vi "ViewAnalysisResults.vi"(7 "LabVIEW Web Service Request":refnum<class "Web Request.lvclass">) -> (3 "Data":T1[](array[typedef]))   [LabVIEW 2019]
uses:
  <vilib>/wsapi/Web Request.lvclass
  ParameterData.ctl
panel:
  # "Use the Web Service Request input terminal to call the VIs on the Web Services palette. Do not remove it from the connector pane unless you don't need access to the palette."
  # "Each additional control wired to the connector pane will be available as an input in the URL. To include an indicator in terminal-mode output (the default setting), it must also be wired to the connector pane."
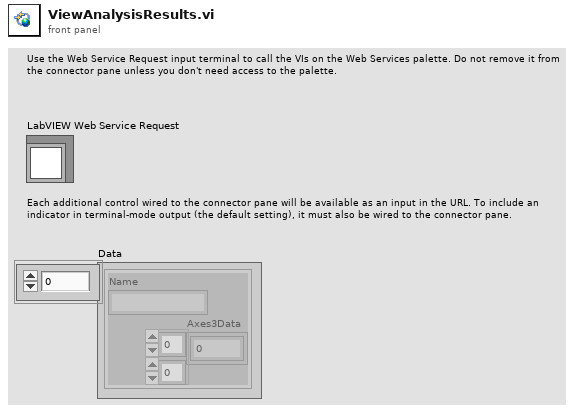
[diagram p1: front panel]
types:
  T1 = typedef "ParameterData.ctl" = cluster{"Name":string, "Axes3Data":dbl[][]}
  T2 = enum16{"open", "open or create", "create or replace", "create", "open (read-only)"}
  T3 = enum16{"open", "replace", "create", "open or create", "replace or create", "replace or create with confirmation"}
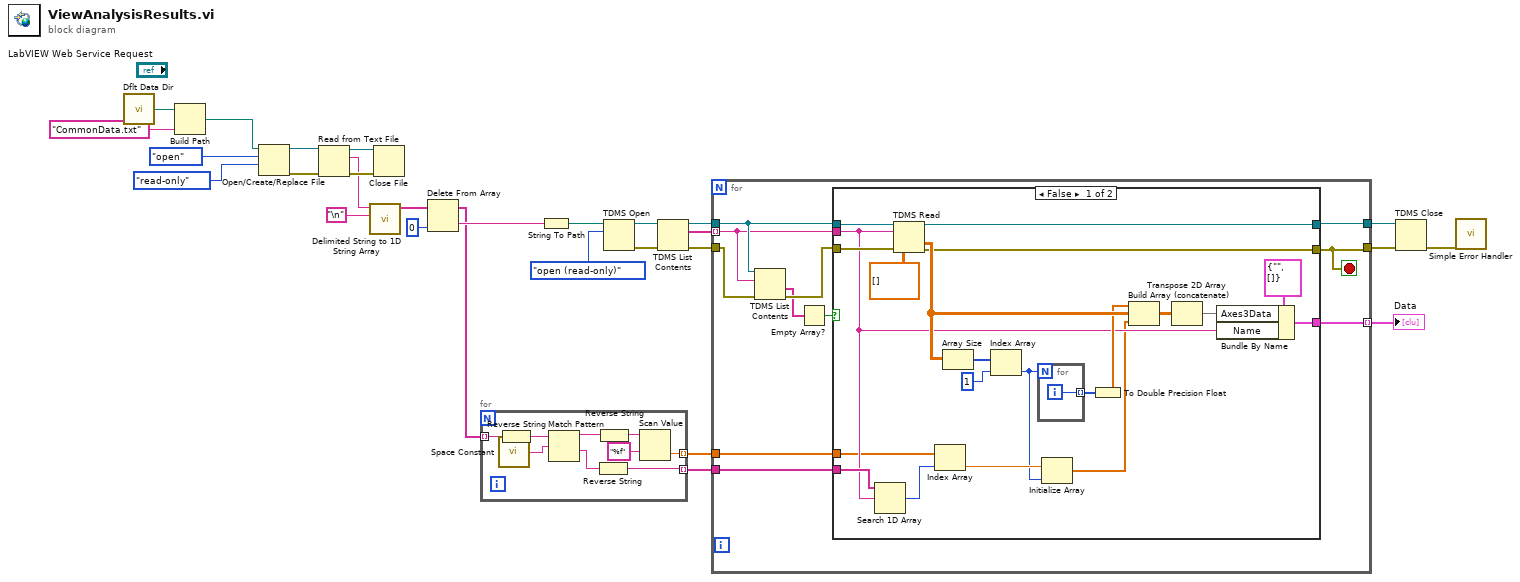
[diagram p0: block diagram]
diagram:
  n1 = call <vilib>:"Dflt Data Dir.vi"() -> ("App:Default Data Directory"=w28:path)
  n2 = Build Path(base path=w28, name or relative path="CommonData.txt") -> (appended path=w26:path)
  n3 = Open/Create/Replace File(file path (use dialog)=w26, operation (0:open)=T3."open", access (0:read/write)=enum16{"read/write", "read-only", "write-only"}."read-only") -> (refnum out=w23:refnum<file>, error out=w22:errorcluster)  [unwired: 3 in, 1 out]
  n4 = Read from Text File(file (use dialog)=w23, error in=w22) -> (refnum out=w21:refnum<file>, text=w8:string, error out=w20:errorcluster)  [unwired: 2 in, 1 out]
  n5 = call <vilib>:"Delimited String to 1D String Array.vi"("delimiter"="\n", "delimited string"=w8) -> ("string array"=w6:string[])  [unwired: 9 in]
  n6 = Close File(refnum=w21, error in=w20) -> ()  [unwired: 2 out]
  n7 = Delete From Array(array=w6, index=0) -> (deleted portion=w4:string, array with subset deleted=w3:string[])  [unwired: 1 in]
  n8 = for {
    tunnel: w3 -> [w37] mode=indexing
    tunnel: [w32] -> w1 mode=indexing
    tunnel: [w29] -> w2 mode=indexing
    n9 = call <vilib>:"Space Constant.vi"() -> ("String"=w35:string)
    n10 = Reverse String(1:w37) -> (0:w36:string)
    n11 = Match Pattern(string=w36, regular expression=w35) -> (before substring=w34:string, after substring=w33:string)  [unwired: 1 in, 2 out]
    n12 = Reverse String(1:w33) -> (0:w32:string)
    n13 = Reverse String(1:w34) -> (0:w31:string)
    n14 = Scan Value(string=w31, format string="%f") -> (value=w29:dbl)  [unwired: 1 in, 1 out]
  }
  n15 = String To Path(string=w4) -> (path=w19:path)
  n16 = TDMS Open(10:T2."open (read-only)" ("operation (0:open)"), 11:w19) -> (0:w16:errorcluster, 3:w17:refnum<k34>)  [unwired: 5 in]
  n17 = TDMS List Contents(4:w16, 7:w17) -> (0:w13:errorcluster, 2:w14:string[], 3:w15:refnum<k34>)  [unwired: 1 in, 1 out]
  n18 = for {
    tunnel: w15 -> [w43]
    tunnel: w14 -> [w42] mode=indexing
    tunnel: w13 -> [w45]
    tunnel: [w48] -> w12
    tunnel: [w46] -> w11
    tunnel: [w47] -> w9 mode=indexing
    tunnel: w2 -> [w39]
    tunnel: w1 -> [w38]
    stop <- w46 stop-if-true
    n19 = TDMS List Contents(4:w45, 6:w42, 7:w43) -> (0:w44:errorcluster, 1:w40:string[])  [unwired: 2 out]
    n20 = Empty Array?(array=w40) -> (empty?=w41:bool)
    n21 = case shown="False" w41 {
      tunnel: w43 -> [w69 w72]
      tunnel: w44 -> [w68 w71]
      tunnel: [w66 w72] -> w48
      tunnel: w42 -> [w54 _]
      tunnel: [w64 _] -> w47
      tunnel: [w57 w71] -> w46
      tunnel: w39 -> [w53 _]
      tunnel: w38 -> [w55 _]
      frame False {
        n22 = Search 1D Array(1D array=w55, element=w54) -> (index of element=w52:i32)  [unwired: 1 in]
        n23 = TDMS Read(0:w69, 5:w54, 11:w68, 12:dbl[][] []) -> (4:w66:refnum<k34>, 10:w59:dbl[][], 15:w57:errorcluster)  [unwired: 4 in, 3 out]
        n24 = Index Array(array=w53, index=w52) -> (element=w51:dbl)
        n25 = Array Size(array=w59) -> (size(s)=w63:i32[])
        n26 = Index Array(array=w63, index=1) -> (element=w50:i32)
        n27 = for {
          N: w50 -> [_]
          tunnel: [w70] -> w61 mode=indexing
          i -> [w70]
        }
        n28 = Initialize Array(w51, w50) -> (w49:dbl[])
        n29 = To Double Precision Float(number=w61) -> (double precision float=w58:dbl[])
        n30 = Build Array (concatenate)(w58, w59, w49) -> (w60:dbl[][])
        n31 = Transpose 2D Array(2D array=w60) -> (transposed array=w56:dbl[][])
        n32 = Bundle By Name(cluster=T1 {"Name"="", "Axes3Data"=[]} ("Parameter"), "Axes3Data"=w56, "Name"=w54) -> (w64:T1)
      }
      frame True {
      }
    }
  }
  "Data" <- w9
  n33 = TDMS Close(8:w11, 11:w12) -> (0:w10:errorcluster)  [unwired: 1 out]
  n34 = call <vilib>:"Simple Error Handler.vi"("error in (no error)"=w10) -> ()  [unwired: 4 in, 5 out]
